vi "mapData.vi"(6 "Zero Index":bool=TRUE, 10 "MAP":string[][](array[string]), 11 "1D Data":dbl[](array[numeric])) -> (3 "Real Matrix":T1)   [LabVIEW 2017]
uses:
  <vilib>/silver_ctls/ArrayMatrixCluster/Real Matrix NI_Silver.ctl
  <vilib>/Analysis/baseanly.llb/Mean (DBL).vi
  <vilib>/Analysis/NI_AALBase.lvlib
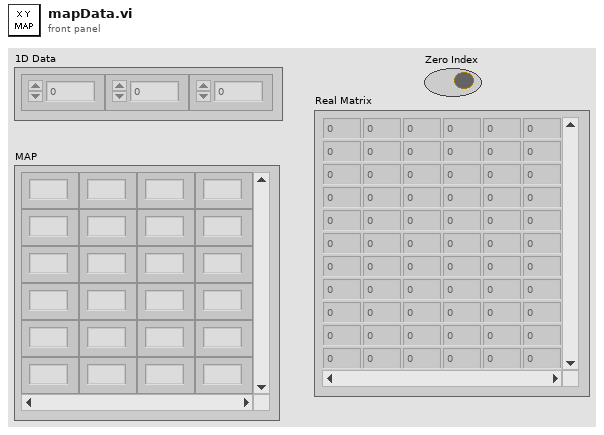
[diagram p1: front panel]
types:
  T1 = typedef "Real Matrix NI_Silver.ctl" = dbl[][]
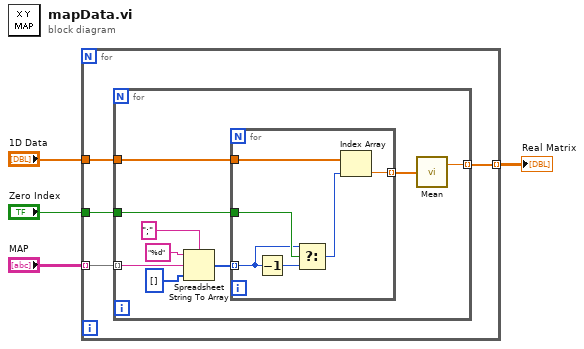
[diagram p0: block diagram]
diagram:
  n1 = for {
    tunnel: "MAP" -> [w8] mode=indexing
    tunnel: "1D Data" -> [w7]
    tunnel: [w6] -> w2 mode=indexing
    tunnel: "Zero Index" -> [w5]
    n2 = for {
      tunnel: w8 -> [w16] mode=indexing
      tunnel: w7 -> [w13]
      tunnel: [w10] -> w6 mode=indexing
      tunnel: w5 -> [w9]
      n3 = Spreadsheet String To Array(delimiter (Tab)=";", format string="%d", spreadsheet string=w16, array type (2D Dbl)=i32[] [] ("1D Data")) -> (array=w12:i32[])
      n4 = for {
        tunnel: w13 -> [w23]
        tunnel: w12 -> [w19] mode=indexing
        tunnel: [w22] -> w11 mode=indexing
        tunnel: w9 -> [w21]
        n5 = Decrement(x=w19) -> (x-1=w20:i32)
        n6 = Select(t=w19, s=w21, f=w20) -> (s? t:f=w18:i32)
        n7 = Index Array(array=w23, index=w18) -> (element=w22:dbl)
      }
      n8 = call-poly <vilib>:"Mean.vi"("X"=w11) -> ("mean"=w10:dbl)  [unwired: 1 out]
    }
  }
  "Real Matrix" <- w2
